vi "TSDC-meas.vi"() -> ()   [LabVIEW 2013]
uses:
  <vilib>/Instr/_visa.llb/VISA Configure Serial Port (Instr).vi
  <vilib>/Utility/file.llb/Write To Spreadsheet File (DBL).vi
panel:
  in  "Chose File (.txt)":path
  in  "Start":bool
  out "Current vs time":cluster{"Y":dbl[], "Y":dbl[]}[](graph) caption="XY Graph"
  out "Current vs Temp":cluster{"Y":dbl[], "Y":dbl[]}[](graph) caption="XY Graph"
  out "read buffer from omega":string
  in  "COM1":refnum<visa-resource-name>="COM1"
  out "Temperature (C)":dbl
  out "Elapsed Time (min)":dbl caption="Elapsed Time (s)"
  out "Current (A)":dbl
  in  "stop":bool
  in  "VISA Resource Name GPIB0::26::INSTR":refnum<visa-resource-name>="GPIB0::2::INSTR"
  out "Read Buffer from electrometer":string
  # "Instrument Address"
  # "Measured Data"
  # "Just a cross check!"
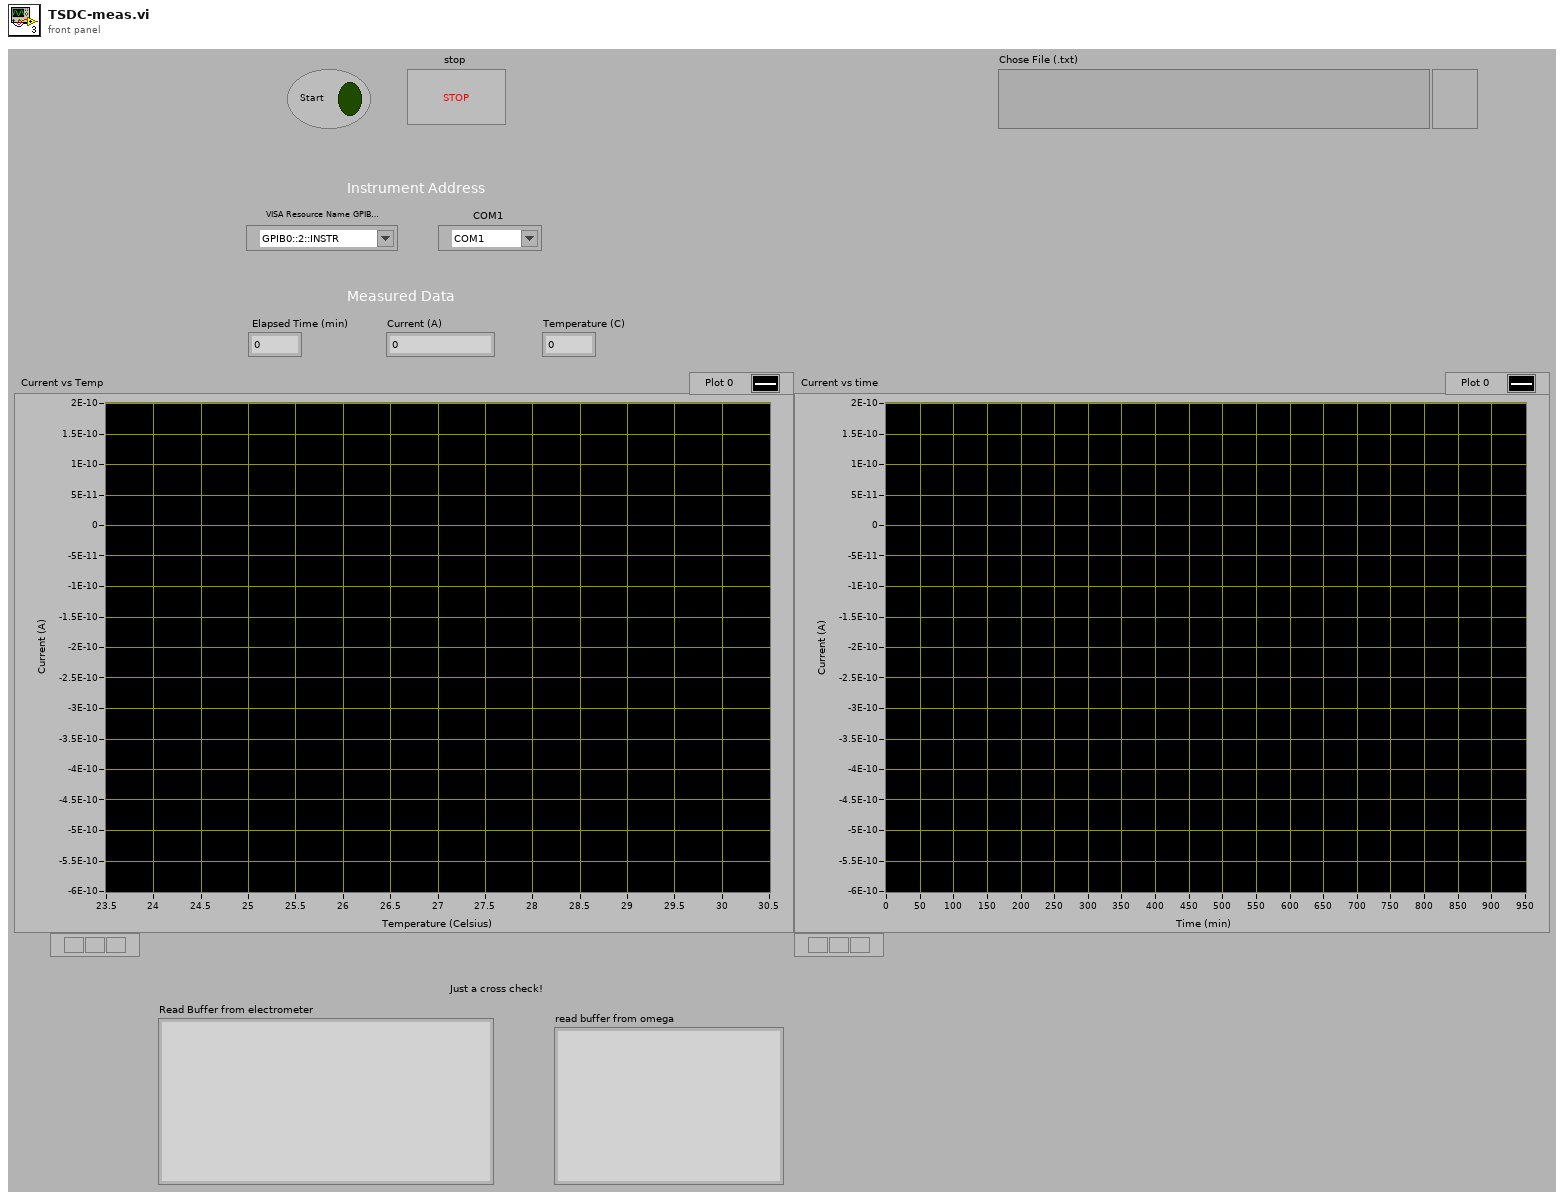
[diagram p1: front panel]
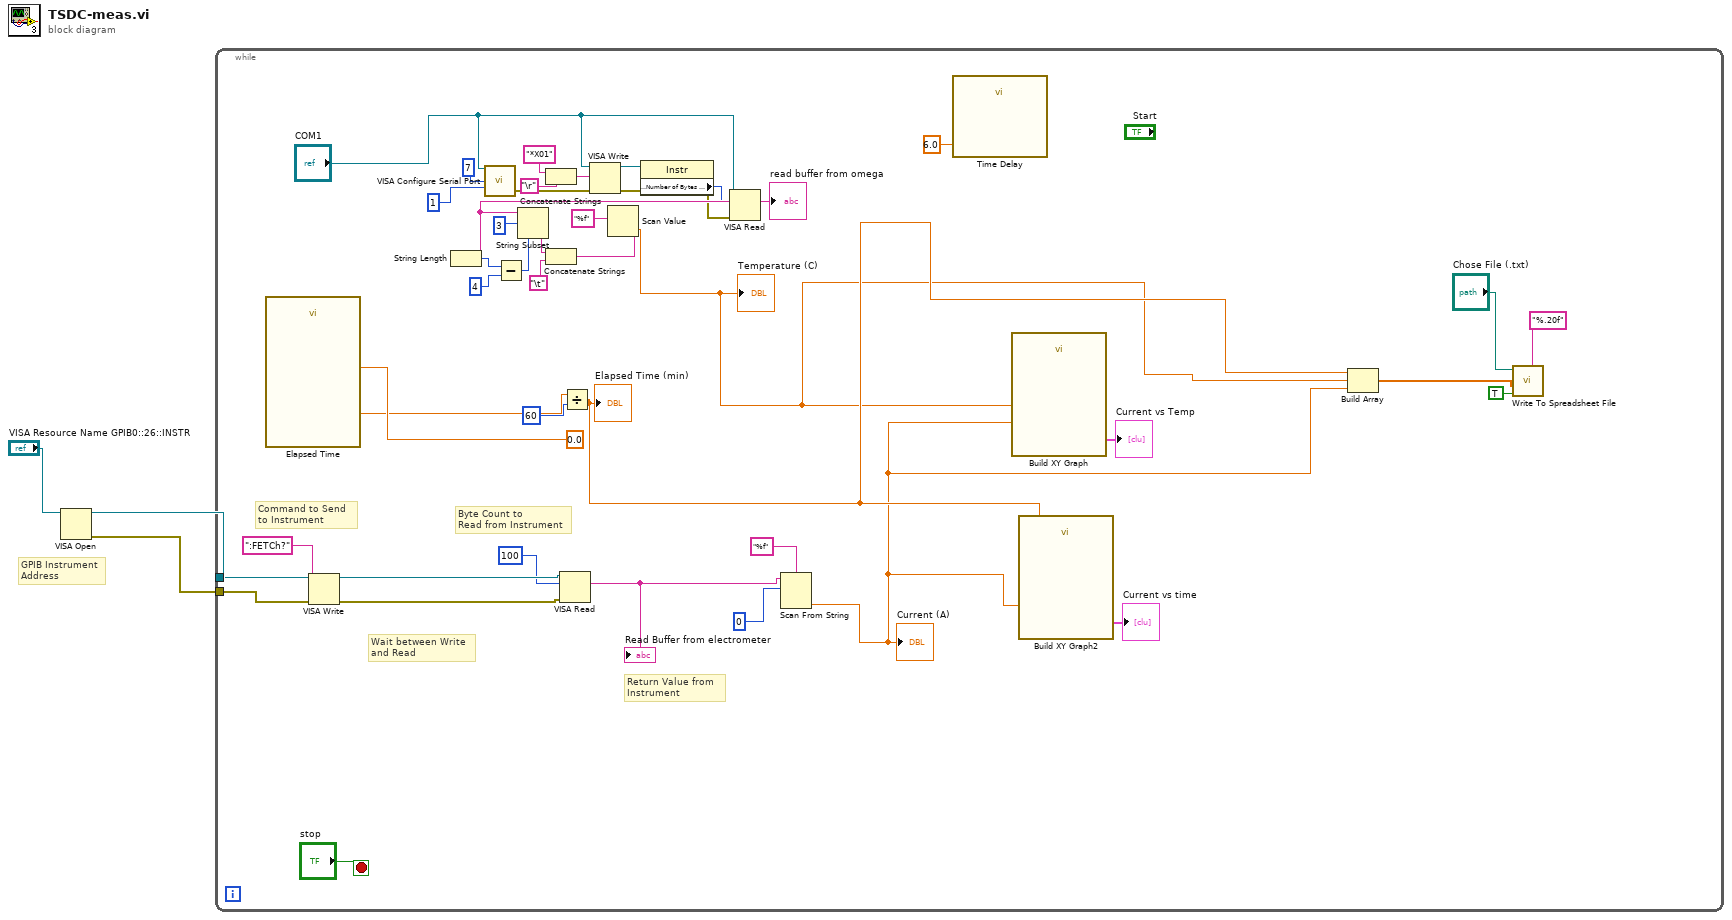
[diagram p0: block diagram]
diagram:
  # "GPIB Instrument\nAddress"
  n1 = VISA Open(VISA resource name="VISA Resource Name GPIB0::26::INSTR") -> (VISA resource name=w1:refnum<visa-resource-name>, error out=w2:errorcluster)  [unwired: 4 in]
  n2 = while {
    tunnel: w2 -> [w45]
    tunnel: w1 -> [w44]
    stop <- "stop" stop-if-true
    # "Wait between Write\nand Read"
    # "Return Value from \nInstrument"
    # "Byte Count to\nRead from Instrument"
    # "Command to Send \nto Instrument"
    n3 = call "Elapsed Time"("Set Start Time (s)"=0.0) -> ("Elapsed Time (s)"=w35:dbl)  [unwired: 11 in, 7 out]
    n4 = VISA Write(VISA resource name=w44, write buffer=":FETCh?" ("Write Buffer"), error in (no error)=w45) -> (VISA resource name out=w42:refnum<visa-resource-name>, error out=w41:errorcluster)  [unwired: 1 out]
    n5 = call-poly "VISA Configure Serial Port"("VISA resource name"="COM1", "data bits (8)"=7, "parity (0:none)"=1) -> ("error out"=w19:errorcluster)  [unwired: 11 in, 1 out]
    n6 = Concatenate Strings("*X01", "\r") -> (w22:string)
    n7 = VISA Read(VISA resource name=w42, byte count=u32 100, error in (no error)=w41) -> (read buffer=w39:string)  [unwired: 3 out]
    "Read Buffer from electrometer" <- w39
    n8 = Divide(x=w35, y=u32 60) -> (x/y=w10:dbl)
    "Elapsed Time (min)" <- w10
    n9 = VISA Write(VISA resource name="COM1", write buffer=w22, error in (no error)=w19) -> (VISA resource name out=w33:refnum<visa-resource-name>, error out=w23:errorcluster)  [unwired: 1 out]
    n10 = property class="Instr"(reference=w33, error in=w23) -> (error out=w24:errorcluster, "Serial Settings:Number of Bytes at Serial Port"=w25:u32)  [unwired: 1 out]
    n11 = VISA Read(VISA resource name="COM1", byte count=w25, error in (no error)=w24) -> (read buffer=w26:string)  [unwired: 3 out]
    "read buffer from omega" <- w26
    n12 = String Length(string=w26) -> (length=w28:i32)
    n13 = Subtract(x=w28, y=4) -> (x-y=w30:i32)
    n14 = String Subset(string=w26, offset (0)=3, length (rest)=w30) -> (substring=w31:string)
    n15 = Concatenate Strings(w31, "\t") -> (w15:string)
    n16 = Scan Value(string=w15, format string="%f") -> (value=w9:dbl)  [unwired: 1 in, 1 out]
    "Temperature (C)" <- w9
    n17 = Scan From String(format string="%f", input string=w39, initial scan location=u32 0) -> (output 1=w8:dbl)  [unwired: 2 in, 3 out]
    "Current (A)" <- w8
    n18 = call "Time Delay"("Delay Time (s)"=6.0) -> ()  [unwired: 10 in, 1 out]
    n19 = call "Build XY Graph"("Y Input"=w8, "X Input"=w9) -> ("XY Graph"=→"Current vs Temp":cluster{"Y":dbl[], "Y":dbl[]}[])  [unwired: 8 in, 1 out]
    n20 = call "Build XY Graph2"("Y Input"=w8, "X Input"=w10) -> ("XY Graph"=→"Current vs time":cluster{"Y":dbl[], "Y":dbl[]}[])  [unwired: 8 in, 1 out]
    n21 = Build Array(w10, w9, w8) -> (w7:dbl[])
    n22 = call-poly <vilib>:"Write To Spreadsheet File.vi"("format (%.3f)"="%.20f", "append to file? (new file:F)"=TRUE, "1D data"=w7, "file path (dialog if empty)"="Chose File (.txt)") -> ()  [unwired: 4 in, 1 out]
  }
